vi "SubPolishVision.vi"() -> (1 "Vison State":bool, 3 "Refnum out":T1)   [LabVIEW 2015]
uses:
  <vilib>/vision/driver/NI_Vision_Acquisition_Software.lvlib
  <vilib>/userdefined/High Color/IMAQdx.ctl
  <vilib>/vision/NI_Vision_Development_Module.lvlib
  <vilib>/vision/Image Controls.llb/IMAQ Image.ctl
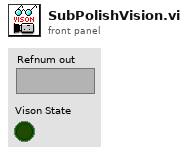
[diagram p1: front panel]
types:
  T1 = typedef "IMAQ Image.ctl" = refnum<image>
  T2 = typedef "IMAQdx.ctl" = refnum<k21>
  T3 = typedef "Image Type" = u32
  T4 = cluster{"Position":cluster{"X":sgl, "Y":sgl}, "Radius":dbl, "Score":dbl}[]
  T5 = cluster{"Circles[0]":cluster{"Position":cluster{"X":sgl, "Y":sgl}, "Radius":dbl, "Score":dbl}, "Circles[1]":cluster{"Position":cluster{"X":sgl, "Y":sgl}, "Radius":dbl, "Score":dbl}, "Circles[2]":cluster{"Position":cluster{"X":sgl, "Y":sgl}, "Radius":dbl, "Score":dbl}, "Circles[3]":cluster{"Position":cluster{"X":sgl, "Y":sgl}, "Radius":dbl, "Score":dbl}, "Circles[4]":cluster{"Position":cluster{"X":sgl, "Y":sgl}, "Radius":dbl, "Score":dbl}, "Circles[5]":cluster{"Position":cluster{"X":sgl, "Y":sgl}, "Radius":dbl, "Score":dbl}, "Circles[6]":cluster{"Position":cluster{"X":sgl, "Y":sgl}, "Radius":dbl, "Score":dbl}, "Circles[7]":cluster{"Position":cluster{"X":sgl, "Y":sgl}, "Radius":dbl, "Score":dbl}, "Circles[8]":cluster{"Position":cluster{"X":sgl, "Y":sgl}, "Radius":dbl, "Score":dbl}}
  T6 = cluster{"Origin Pixel":cluster{"X":sgl, "Y":sgl}, "X Axis Pixel":cluster{"X":sgl, "Y":sgl}, "Axis Reference":u32}
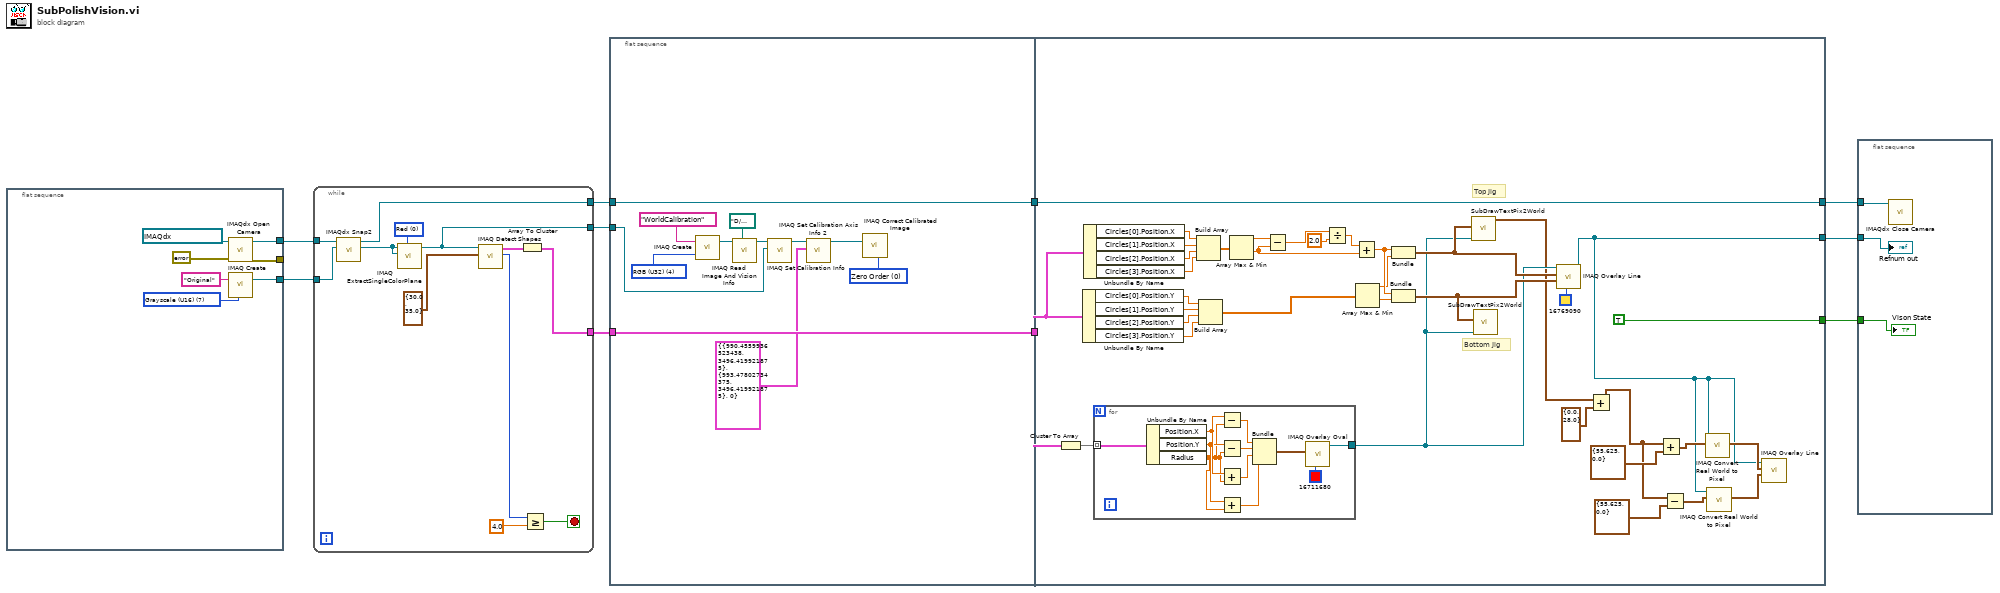
[diagram p0: block diagram]
diagram:
  n1 = flat-sequence {
    tunnel: [w13] -> w10
    tunnel: [w12] -> w9
    tunnel: [w11] -> _
    frame #0 {
      w15 = T3 7 items=["Grayscale (U8)", "Grayscale (I16)", "Grayscale (SGL)", "Complex (CSG)", "RGB (U32)", "HSL (U32)", "RGB (U64)", "Grayscale (U16)"] ("Image Type")
      n2 = call <vilib>:"IMAQdx Open Camera.vi"("error in"=errorcluster {"status"=FALSE, "code"=0, "source"=""}, "Session In"=T2 "acA1920-25gc") -> ("error out"=w11:errorcluster, "Session Out"=w13:T2)  [unwired: 8 in]
      n3 = call "IMAQ Create"("Image Name"="Original", "Image Type"=w15) -> ("New Image"=w12:T1)  [unwired: 3 in, 1 out]
    }
  }
  n4 = while {
    tunnel: w10 -> [w29]
    tunnel: w9 -> [w28]
    tunnel: [w20] -> w8
    tunnel: [w19] -> w7
    tunnel: [w18] -> w6
    stop <- w21 stop-if-true
    w27 = 0 items=["Red", "Green", "Blue", "Hue", "Saturation", "Luminance", "Value", "Intensity"] ("Color Plane")
    n5 = call <vilib>:"IMAQdx Snap2.vi"("Image In"=w28, "Session In"=w29) -> ("Image Out"=w26:T1, "Session Out"=w18:T2)  [unwired: 7 in, 1 out]
    n6 = call "IMAQ ExtractSingleColorPlane"("Color Plane"=w27, "Image Dst"=w26, "Image Src"=w26) -> ("Image Dst Out"=w19:T1)  [unwired: 7 in, 1 out]
    n7 = call-poly "IMAQ Detect Shapes"("Circle Descriptor"=cluster{"Min Radius":dbl, "Max Radius":dbl} {"Min Radius"=30.0, "Max Radius"=35.0}, "Image"=w19) -> ("Number of Matches Returned"=w22:i32, "Circles"=w23:T4)  [unwired: 7 in, 1 out]
    n8 = Array To Cluster(array=w23) -> (cluster=w20:T5)
    n9 = Greater Or Equal?(x=w22, y=4.0) -> (x >= y?=w21:bool)
  }
  n10 = flat-sequence {
    tunnel: w6 -> [w40]
    tunnel: w7 -> [w31]
    tunnel: w8 -> [w41]
    tunnel: [w41] -> w4
    tunnel: [w40] -> w3
    tunnel: w4 -> [w56]
    tunnel: w3 -> [w59]
    tunnel: [w59] -> w5
    tunnel: [TRUE] -> w2
    tunnel: [w43] -> w1
    frame #0 {
      w32 = u32 0 items=["Zero Order", "Bi-Linear", "Quadratic", "Cubic Spline"] ("Interpolation Type")
      w38 = T3 4 items=["Grayscale (U8)", "Grayscale (I16)", "Grayscale (SGL)", "Complex (CSG)", "RGB (U32)", "HSL (U32)", "RGB (U64)", "Grayscale (U16)"] ("Image Type")
      n11 = call "IMAQ Create"("Image Name"="WorldCalibration", "Image Type"=w38) -> ("New Image"=w36:T1)  [unwired: 2 in, 2 out]
      n12 = call "IMAQ Read Image And Vision Info"("File Path"=path "D:/PolishingRobot/LastEdition/config setting/WorldCalibration.png", "Image"=w36) -> ("Image Out"=w39:T1)  [unwired: 2 in, 7 out]
      n13 = call "IMAQ Set Calibration Info"("Image Dst"=w31, "Image Src"=w39) -> ("Calibrated Image"=w33:T1)  [unwired: 2 in, 7 out]
      n14 = call-poly "IMAQ Set Calibration Axis Info 2"("Calibration Axis Info"=T6 {"Origin Pixel"={"X"=990.456, "Y"=3496.42}, "X Axis Pixel"={"X"=993.478, "Y"=3496.42}, "Axis Reference"=0}, "Calibration Template Image In"=w33) -> ("Calibration Template Image Out"=w30:T1)  [unwired: 1 in, 8 out]
      n15 = call "IMAQ Correct Calibrated Image"("Interpolation Type"=w32, "Image Src"=w30) -> ()  [unwired: 5 in, 5 out]
    }
    frame #1 {
      # "Top Jig"
      # "Bottom Jig"
      n16 = Cluster To Array(cluster=w56) -> (array=w57:T4)
      n17 = Unbundle By Name(w56) -> ("Circles[0].Position.Y"=w73:sgl, "Circles[1].Position.Y"=w72:sgl, "Circles[2].Position.Y"=w71:sgl, "Circles[3].Position.Y"=w70:sgl)
      n18 = Unbundle By Name(w56) -> ("Circles[0].Position.X"=w77:sgl, "Circles[1].Position.X"=w76:sgl, "Circles[2].Position.X"=w75:sgl, "Circles[3].Position.X"=w74:sgl)
      n19 = for {
        tunnel: w57 -> [w85] mode=indexing
        tunnel: [w86] -> w52
        n20 = Unbundle By Name(w85) -> ("Position.X"=w83:sgl, "Position.Y"=w81:sgl, "Radius"=w80:dbl)
        n21 = Subtract(x=w83, y=w80) -> (x-y=w84:dbl)
        n22 = Subtract(x=w81, y=w80) -> (x-y=w88:dbl)
        n23 = Add(x=w83, y=w80) -> (x+y=w82:dbl)
        n24 = Add(x=w81, y=w80) -> (x+y=w79:dbl)
        n25 = Bundle(w84, w88, w82, w79) -> (w78:cluster{dbl, dbl, dbl, dbl})  [unwired: 1 in]
        n26 = call "IMAQ Overlay Oval"("Color"=u32 16711680, "Bounding Rectangle"=w78) -> ("Image Out"=w86:T1)  [unwired: 8 in, 1 out]
      }
      n27 = Build Array(w77, w76, w75, w74) -> (w69:sgl[])
      n28 = Build Array(w73, w72, w71, w70) -> (w68:sgl[])
      n29 = Array Max & Min(array=w69) -> (max value=w63:sgl, min value=w58:sgl)  [unwired: 2 out]
      n30 = Subtract(x=w63, y=w58) -> (x-y=w67:sgl)
      n31 = Divide(x=w67, y=sgl 2.0) -> (x/y=w65:sgl)
      n32 = Add(x=w65, y=w58) -> (x+y=w64:sgl)
      n33 = Array Max & Min(array=w68) -> (max value=w62:sgl, min value=w61:sgl)  [unwired: 2 out]
      n34 = Bundle(w64, w62) -> (w54:cluster{sgl, sgl})  [unwired: 1 in]
      n35 = Bundle(w64, w61) -> (w53:cluster{sgl, sgl})  [unwired: 1 in]
      n36 = call "SubDrawTextPix2World.vi"("X Y Pixel Co-Ordinate"=w54, "Refnum Img Out"=w52) -> ("X Y World Co-Ordinate"=w42:cluster{sgl, sgl})  [unwired: 7 in]
      n37 = call "SubDrawTextPix2World.vi"("X Y Pixel Co-Ordinate"=w53, "Refnum Img Out"=w52) -> ()  [unwired: 7 in, 1 out]
      n38 = call "IMAQ Overlay Line"("Color"=u32 16769090, "End Point"=w53, "Start Point"=w54, "Image"=w52) -> ("Image Out"=w43:T1)  [unwired: 6 in, 1 out]
      n39 = Add(x=w42, y=cluster{sgl, sgl} {0.0, 28.0}) -> (x+y=w48:cluster{sgl, sgl})
      n40 = Add(x=w48, y=cluster{sgl, sgl} {55.625, 0.0}) -> (x+y=w47:cluster{sgl, sgl})
      n41 = Subtract(x=w48, y=cluster{sgl, sgl} {55.625, 0.0}) -> (x-y=w46:cluster{sgl, sgl})
      n42 = call "IMAQ Convert Real World to Pixel"("Real World Coordinates"=w47, "Calibrated Image"=w43) -> ("Pixel Coordinates"=w45:cluster{"X":sgl, "Y":sgl})  [unwired: 4 in, 5 out]
      n43 = call "IMAQ Convert Real World to Pixel"("Real World Coordinates"=w46, "Calibrated Image"=w43) -> ("Pixel Coordinates"=w44:cluster{"X":sgl, "Y":sgl})  [unwired: 4 in, 5 out]
      n44 = call "IMAQ Overlay Line"("End Point"=w44, "Start Point"=w45, "Image"=w43) -> ()  [unwired: 7 in, 2 out]
    }
  }
  n45 = flat-sequence {
    tunnel: w5 -> [w91]
    tunnel: w2 -> [w90]
    tunnel: w1 -> [w89]
    frame #0 {
      n46 = call <vilib>:"IMAQdx Close Camera.vi"("Session In"=w91) -> ()  [unwired: 10 in, 1 out]
      "Refnum out" <- w89
      "Vison State" <- w90
    }
  }
